vi "menu-InterleaveSeperators.vi"(11 "Array":cluster{"element":T1[]}[](array[cluster])) -> (3 "element":T1[](array[typedef]))   [LabVIEW 2017, in "menu-operation.lvlib"]
uses:
  menu-operation.lvlib
  <resource>/Framework/Providers/API/mxLvMenuItem.ctl
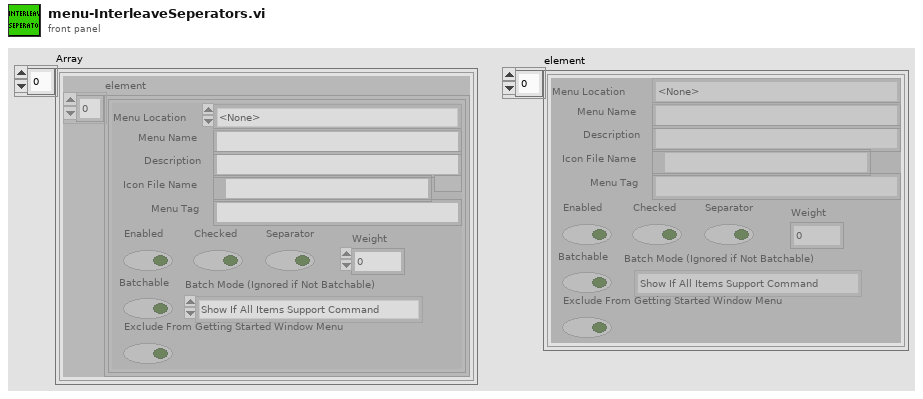
[diagram p1: front panel]
types:
  T1 = typedef "mxLvMenuItem.ctl" = cluster{"Menu Name":string, "Description":string, "Icon File Name":path, "Menu Tag":string, "Enabled":bool, "Checked":bool, "Separator":bool, "Batchable":bool, "Weight":i32, "Batch Mode (Ignored if Not Batchable)":enum32{"Show If All Items Support Command", "Show If Any Items Support Command"}, "Menu Location":enum32{"<None>", "Project", "Project / Build Specifications", "Tools", "Tools / Source Control", "Tools / Real-Time Module", "Help"}, "Exclude From Getting Started Window Menu":bool}
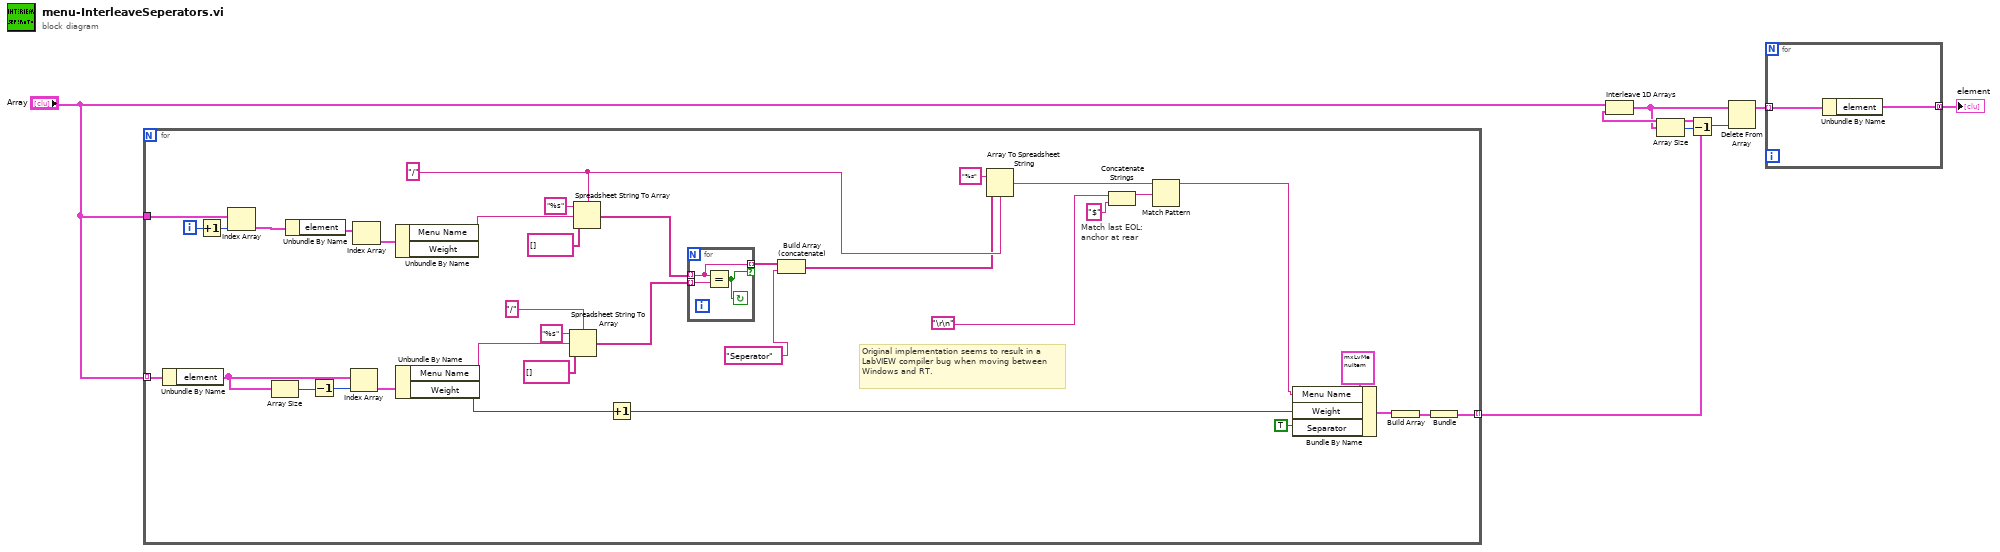
[diagram p0: block diagram]
diagram:
  n1 = for {
    tunnel: "Array" -> [w44] mode=indexing
    tunnel: [w34] -> w5 mode=indexing
    tunnel: "Array" -> [w33]
    i -> [w32]
    w26 = "/" ("delimiter (Tab)")
    # "Original implementation seems to result in a LabVIEW compiler bug when moving between Windows and RT."
    # "Match last EOL:\nanchor at rear"
    n2 = Unbundle By Name(w44) -> ("element"=w43:T1[])
    n3 = Increment(x=w32) -> (x+1=w31:i32)
    n4 = Index Array(array=w33, index=w31) -> (element=w30:cluster{"element":T1[]})
    n5 = Array Size(array=w43) -> (size(s)=w17:i32)
    n6 = Unbundle By Name(w30) -> ("element"=w29:T1[])
    n7 = Decrement(x=w17) -> (x-1=w18:i32)
    n8 = Index Array(array=w43, index=w18) -> (element=w28:T1)
    n9 = Index Array(array=w29) -> (element=w27:T1)  [unwired: 1 in]
    n10 = Unbundle By Name(w27) -> ("Menu Name"=w25:string)  [unwired: 1 out]
    n11 = Unbundle By Name(w28) -> ("Menu Name"=w39:string, "Weight"=w41:i32)
    n12 = Spreadsheet String To Array(delimiter (Tab)="/", format string="%s", spreadsheet string=w39, array type (2D Dbl)=string[] [] ("Array of Strings")) -> (array=w23:string[])
    n13 = Spreadsheet String To Array(delimiter (Tab)=w26, format string="%s", spreadsheet string=w25, array type (2D Dbl)=string[] [] ("Array of Strings")) -> (array=w24:string[])
    n14 = Increment(x=w41) -> (x+1=w40:i32)
    n15 = for {
      tunnel: w24 -> [w46] mode=indexing
      tunnel: w23 -> [w47] mode=indexing
      tunnel: [w46] -> w22 mode=indexing if=w45
      stop <- w45 continue-if-true
      n16 = Equal?(x=w46, y=w47) -> (x = y?=w45:bool)
    }
    n17 = Build Array (concatenate)(w22, "Seperator" ("delimiter (Tab)")) -> (w21:string[])
    n18 = Array To Spreadsheet String(delimiter (Tab)=w26, array=w21, 3:"%s" ("format string")) -> (spreadsheet string=w11:string)
    n19 = Concatenate Strings("\r\n", "$" ("Substring")) -> (w10:string)
    n20 = Match Pattern(string=w11, regular expression=w10) -> (before substring=w20:string)  [unwired: 1 in, 3 out]
    n21 = Bundle By Name(cluster=T1 {"Menu Name"="Seperator", "Description"="", "Icon File Name"=path "", "Menu Tag"="", "Enabled"=TRUE, "Checked"=FALSE, "Separator"=TRUE, "Batchable"=FALSE, "Weight"=0, "Batch Mode (Ignored if Not Batchable)"=enum."Show If All Items Support Command", "Menu Location"=enum."<None>", "Exclude From Getting Started Window Menu"=FALSE} ("Menu Item"), "Menu Name"=w20, "Weight"=w40, "Separator"=TRUE) -> (w36:T1)
    n22 = Build Array(w36) -> (w35:T1[])
    n23 = Bundle(w35) -> (w34:cluster{T1[]})  [unwired: 1 in]
  }
  n24 = Interleave 1D Arrays("Array", w5) -> (w2:cluster{"element":T1[]}[])
  n25 = Array Size(array=w2) -> (size(s)=w4:i32)
  n26 = Decrement(x=w4) -> (x-1=w3:i32)
  n27 = Delete From Array(array=w2, index=w3) -> (array with subset deleted=w6:cluster{"element":T1[]}[])  [unwired: 1 in, 1 out]
  n28 = for {
    tunnel: w6 -> [w49] mode=indexing
    tunnel: [w48] -> w7 mode=concatenating
    n29 = Unbundle By Name(w49) -> ("element"=w48:T1[])
  }
  "element" <- w7
